vi "File Save-DS.vi"(0 "Cancel Button":bool, 8 "error in":errorcluster, 11 "Path":path) -> (1 "Save Button Ind":bool, 2 "error out":errorcluster, 3 "refnum out":refnum<file>, 4 "File Name Ind":string)   [LabVIEW 2020]
panel:
  in  "File Name":string
  in  "Save Button":bool
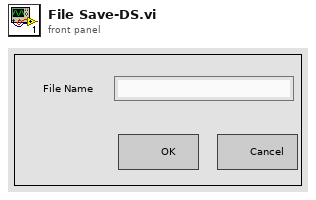
[diagram p1: front panel]
types:
  T1 = enum16{"open", "replace", "create", "open or create", "replace or create", "replace or create with confirmation"}
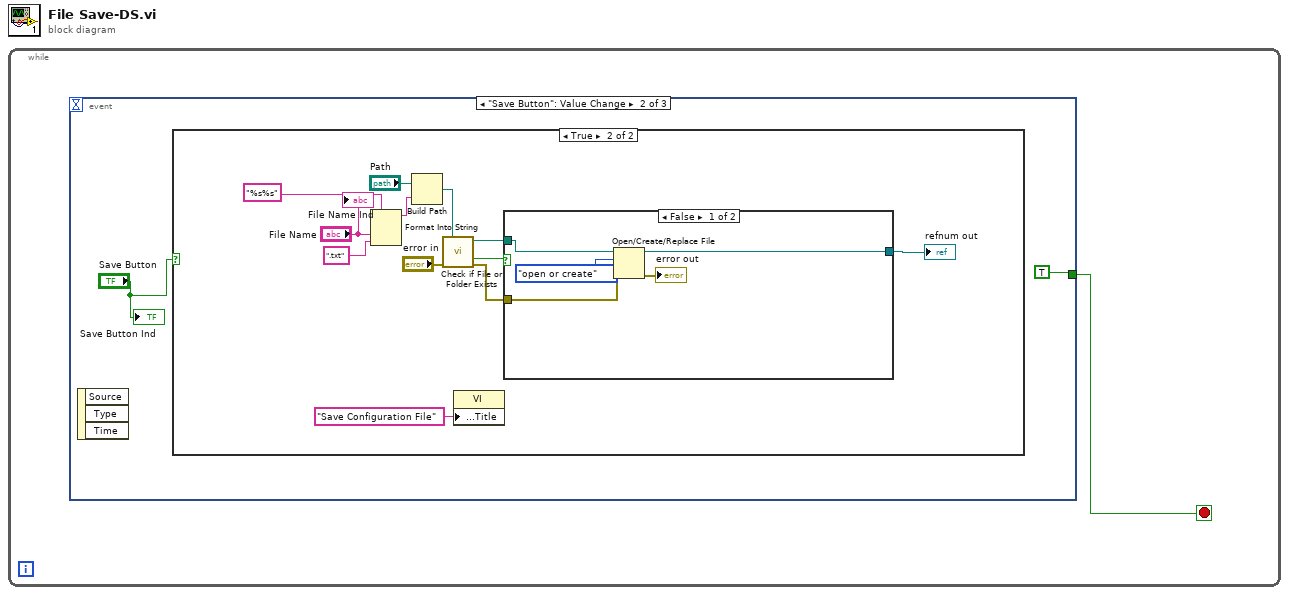
[diagram p0: block diagram]
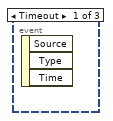
[diagram p2: hidden frame]
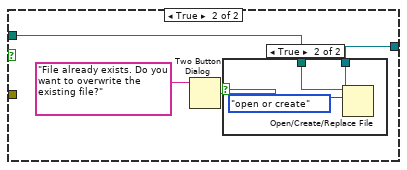
[diagram p4: hidden frame]
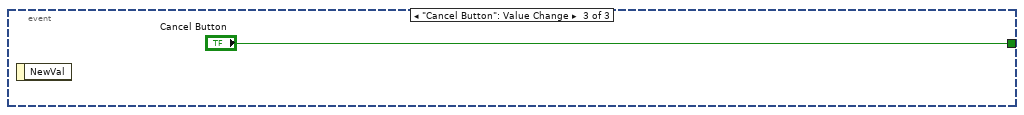
[diagram p6: hidden frame]
diagram:
  n1 = while {
    stop <- w1 stop-if-true
    n2 = event shown="[1] \"Save Button\": Value Change" {
      selector: _ -> [_ _ _]
      dyn-events: _ -> [_ _ _]
      timeout: _ -> [_ _ _]
      tunnel: [_ TRUE ("Cancel Button") "Cancel Button"] -> w1
      event Timeout {
        n3 = event-data() -> ()  [unwired: 1 in, 3 out]
      }
      event "Save Button": Value Change {
        n4 = event-data() -> ()  [unwired: 1 in, 3 out]
        n5 = case shown="True" "Save Button" {
          frame False {
          }
          frame True {
            n6 = Format Into String(format string="%s%s", "File Name", ".txt" ("pattern (all files)")) -> (resulting string=w13:string)  [unwired: 2 in, 1 out]
            n7 = Build Path(base path="Path", name or relative path=w13) -> (appended path=w12:path)
            n8 = call <vilib>:"Check if File or Folder Exists.vi"("error in (no error)"="error in", "path"=w12) -> ("error out"=w10:errorcluster, "file or folder exists?"=w9:bool, "dup path"=w8:path)  [unwired: 7 in]
            n9 = property class="VI"("Front Panel.Title"="Save Configuration File" ("Front Panel Window:Title")) -> ()  [unwired: 2 in, 2 out]
            n10 = case shown="False" w9 {
              tunnel: w10 -> [w20 _]
              tunnel: w8 -> [w17 w22]
              tunnel: [w16 w21] -> w6
              frame False {
                n11 = Open/Create/Replace File(file path (use dialog)=w17, error in=w20, operation (0:open)=T1."open or create") -> (refnum out=w16:refnum<file>, error out=→"error out":errorcluster)  [unwired: 3 in, 1 out]
              }
              frame True {
                n12 = Two Button Dialog(message="File already exists. Do you want to overwrite the existing file?") -> (T button?=w23:bool)  [unwired: 2 in]
                n13 = case shown="True" w23 {
                  tunnel: w22 -> [_ w27]
                  tunnel: [_ w26] -> w21
                  frame False {
                  }
                  frame True {
                    n14 = Open/Create/Replace File(file path (use dialog)=w27, operation (0:open)=T1."open or create") -> (refnum out=w26:refnum<file>)  [unwired: 4 in, 2 out]
                  }
                }
              }
            }
            "refnum out" <- w6
            "File Name Ind" <- "File Name"
          }
        }
        "Save Button Ind" <- "Save Button"
      }
      event "Cancel Button": Value Change {
        n15 = event-data() -> ()  [unwired: 1 in, 1 out]
      }
    }
  }
